vi "LF End Of File__ogtk.vi"(4 "error in (no error)":errorcluster, 5 "offset in (0)":dbl, 6 "pos mode (end)":enum16{"start", "end", "current"}(ring)=enum."end", 7 "refnum":refnum<file>) -> (0 "error out":errorcluster, 1 "offset out":dbl, 3 "refnum out":refnum<file>)   [LabVIEW 2014]
doc: "Changes the size of a file as double float to work for files larger than 2GB."
panel:
  # "LF  End Of File.vi\n\nPlease visit http://www.OpenG.org to learn about the\nOpen Source LabVIEW software movement.\n\nNOTICE -- YOU MUST LEAVE THIS NOTICE IN PLACE.  PER THE TERMS OF THE LICENSE BELOW, YOU MAY SUBLICENSE THIS SOFTWARE \nIN ANY WAY THAT DOES NOT CONFLICT WITH THIS LICENSE.\n\n### BSD License (http://www.opensource.org/licenses/bsd-license.php) Begin ###\n\nCopyright (c) 2003, Rolf Kalbermatter <rolf.kalbermatter@citeng.com>\n\nAll rights reserved.\n\nRedistribution and use in source and binary forms, with or without modification, are permitted provided that the following conditions are met:\n\n    * Redistributions of source code must retain the above copyright notice, this list of conditions and the following disclaimer.\n    * Redistributions in binary form must reproduce the above copyright notice, this list of conditions and the following disclaimer in the \n       documentation and/or other materials provided with the distribution.\n    * Neither the name of SciWare, James Kring, Inc., nor the names of its contributors may be used to endorse or promote products derived \n       from this software without specific prior written permission.\n\nTHIS SOFTWARE IS PROVIDED BY THE COPYRIGHT HOLDERS AND CONTRIBUTORS \"AS IS\" AND ANY EXPRESS OR IMPLIED WARRANTIES, \nINCLUDING, BUT NOT LIMITED TO, THE IMPLIED WARRANTIES OF MERCHANTABILITY AND FITNESS FOR A PARTICULAR PURPOSE ARE \nDISCLAIMED. IN NO EVENT SHALL THE COPYRIGHT OWNER OR CONTRIBUTORS BE LIABLE FOR ANY DIRECT, INDIRECT, INCIDENTAL,\n SPECIAL, EXEMPLARY, OR CONSEQUENTIAL DAMAGES (INCLUDING, BUT NOT LIMITED TO, PROCUREMENT OF SUBSTITUTE GOODS OR \nSERVICES; LOSS OF USE, DATA, OR PROFITS; OR BUSINESS INTERRUPTION) HOWEVER CAUSED AND ON ANY THEORY OF LIABILITY, \nWHETHER IN CONTRACT, STRICT LIABILITY, OR TORT (INCLUDING NEGLIGENCE OR OTHERWISE) ARISING IN ANY WAY OUT OF THE USE \nOF THIS SOFTWARE, EVEN IF ADVISED OF THE POSSIBILITY OF SUCH DAMAGE.\n\n### BSD License End ###"
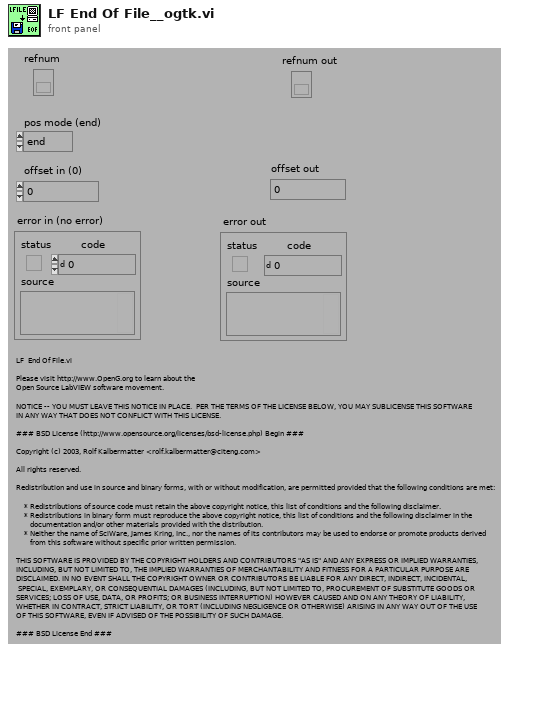
[diagram p1: front panel]
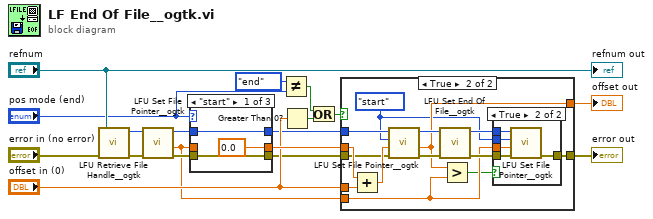
[diagram p0: block diagram]
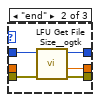
[diagram p4: hidden frame]
diagram:
  n1 = call <userlib>:"LFU Retrieve File Handle__ogtk.vi"("error in (no error)"="error in (no error)", "file refnum"="refnum") -> ("error out"=w3:errorcluster, "handle out"=w2:u32)  [unwired: 4 in]
  n2 = call <userlib>:"LFU Set File Pointer__ogtk.vi"("error in (no error)"=w3, "handle"=w2) -> ("error out"=w4:errorcluster, "offset out"=w1:dbl, "handle out"=w5:u32)  [unwired: 3 in]
  n3 = case shown="\"start\"" "pos mode (end)" {
    tunnel: [w19 w26 w27] -> w7
    tunnel: [0.0 ("offset out") w24 w28] -> w16
    tunnel: [w20 w25 w29] -> w6
    tunnel: w5 -> [w20 w23 w29]
    tunnel: w1 -> [_ _ w28]
    tunnel: w4 -> [w19 w22 w27]
    frame "start" {
    }
    frame "end" {
      n4 = call <userlib>:"LFU Get File Size__ogtk.vi"("error in (no error)"=w22, "handle"=w23) -> ("error out"=w26:errorcluster, "file size"=w24:dbl, "handle out"=w25:u32)  [unwired: 3 in]
    }
    frame "current" {
    }
  }
  n5 = Not Equal?(x=enum16{"start", "end", "current"}."end", y="pos mode (end)") -> (x != y?=w10:bool)
  n6 = Greater Than 0?(x="offset in (0)") -> (x > 0?=w11:bool)
  n7 = Or(x=w10, y=w11) -> (x .or. y?=w13:bool)
  n8 = case shown="True" w13 {
    tunnel: w16 -> [w31 w45]
    tunnel: "offset in (0)" -> [_ w44]
    tunnel: w7 -> [w30 w36]
    tunnel: [w30 w38] -> w15
    tunnel: [w31 w35] -> w14
    tunnel: w6 -> [_ w37]
    tunnel: w1 -> [_ w34]
    frame False {
    }
    frame True {
      w32 = enum16{"start", "end", "current"}."start" ("pos mode (current)")
      n9 = Add(x=w45, y=w44) -> (x+y=w43:dbl)
      n10 = call <userlib>:"LFU Set File Pointer__ogtk.vi"("error in (no error)"=w36, "offset in (0)"=w43, "pos mode (current)"=w32, "handle"=w37) -> ("error out"=w42:errorcluster, "offset out"=w35:dbl, "handle out"=w41:u32)  [unwired: 1 in]
      n11 = call <userlib>:"LFU Set End Of File__ogtk.vi"("error in (no error)"=w42, "handle"=w41) -> ("error out"=w40:errorcluster, "handle out"=w39:u32)  [unwired: 4 in]
      n12 = Greater?(x=w35, y=w34) -> (0:w33:bool)
      n13 = case shown="True" w33 {
        tunnel: w40 -> [w46 w51]
        tunnel: w39 -> [_ w50]
        tunnel: [w46 w49] -> w38
        tunnel: w34 -> [_ w48]
        tunnel: w32 -> [_ w47]
        frame False {
        }
        frame True {
          n14 = call <userlib>:"LFU Set File Pointer__ogtk.vi"("error in (no error)"=w51, "offset in (0)"=w48, "pos mode (current)"=w47, "handle"=w50) -> ("error out"=w49:errorcluster)  [unwired: 1 in, 2 out]
        }
      }
    }
  }
  "error out" <- w15
  "offset out" <- w14
  "refnum out" <- "refnum"
